vi "Get Failure Action Event.vi"(8 "error in (no error)":errorcluster, 10 "Assert VI UID":i32) -> (0 "error out":errorcluster, 3 "Failure Action Event References":T1)   [LabVIEW 2016, in "Assert API Components.lvlib" / "Log Assert Core.lvlib"]
uses:
  Log Assert Core.lvlib
  Failure Action Change Event Reference.ctl
  Failure Actions.ctl
  Assert API Components.lvlib
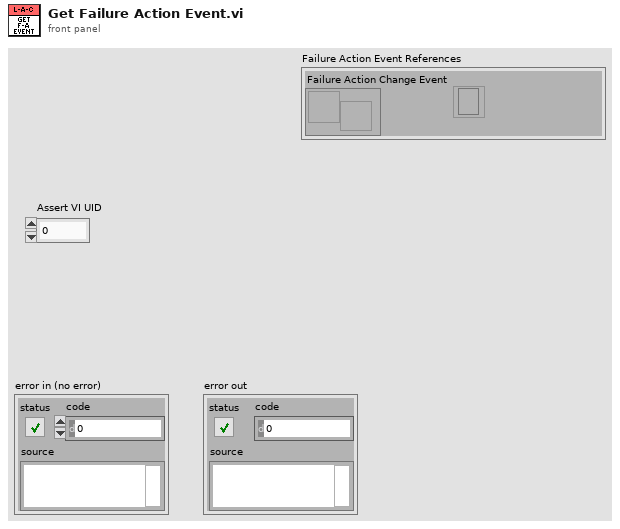
[diagram p1: front panel]
types:
  T1 = typedef "Assert API Components.lvlib/Log Assert Core.lvlib/Failure Action Change Event Reference.ctl" = cluster{"Failure Action Change Event":refnum<user-event>, "Event Registration Refnum":refnum<event-registration>}
  T2 = typedef "Assert API Components.lvlib/Failure Actions.ctl" = enum16{"None", "Log To File", "Pause Execution", "Abort Execution"}
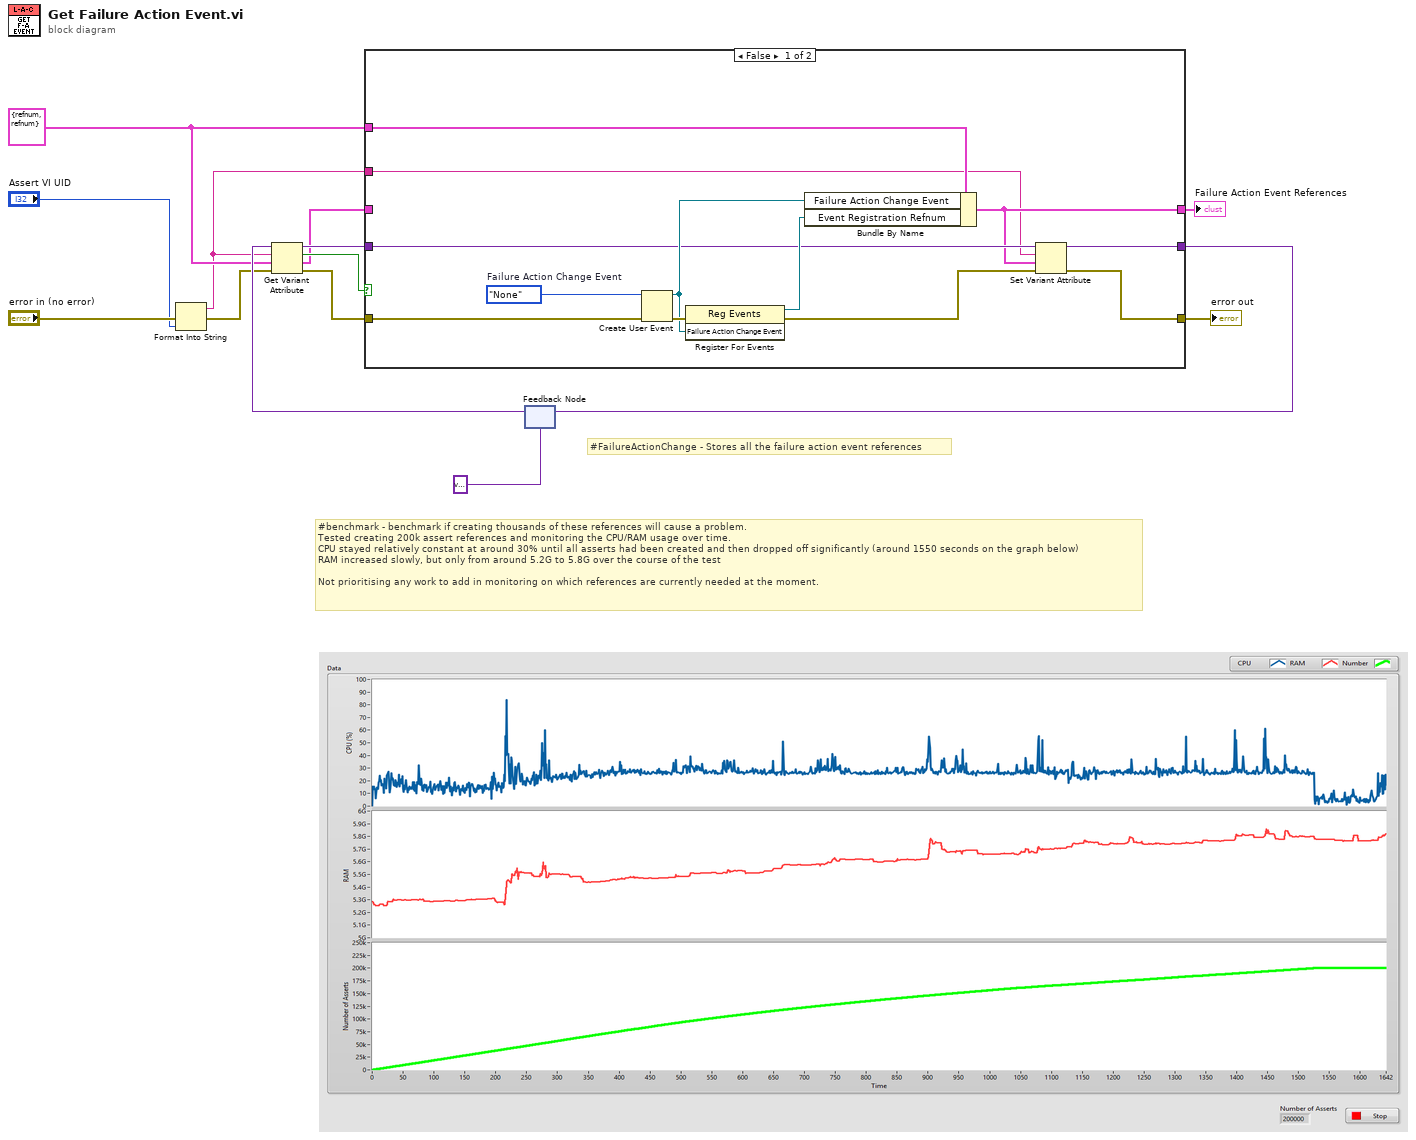
[diagram p0: block diagram]
diagram:
  w5 = T1 {"Failure Action Change Event"=refnum, "Event Registration Refnum"=refnum} ("Cluster")
  # "#benchmark - benchmark if creating thousands of these references will cause a problem. \nTested creating 200k assert references and monitoring the CPU/RAM usage over time.\nCPU stayed relatively constant at around 30% until all asserts had been created and then dropped off significantly (around 1550 seconds on the graph below)\nRAM increased slowly, but only from around 5.2G to 5.8G over the course of the test\n\nNot prioritising any work to add in monitoring on which references are currently needed at the moment."
  # "#FailureActionChange - Stores all the failure action event references"
  n1 = Format Into String(error in="error in (no error)", "Assert VI UID") -> (resulting string=w2:string, error out=w7:errorcluster)  [unwired: 2 in]
  n2 = feedback #1(variant) -> (w11:variant)
  n3 = Get Variant Attribute(Variant=w11, name=w2, default value (empty Variant)=w5, error in=w7) -> (duplicate Variant=w10:variant, found=w4:bool, value=w3:T1, error out=w8:errorcluster)
  n4 = case shown="False" w4 {
    tunnel: [w19 w29] -> w14
    tunnel: w8 -> [w25 w29]
    tunnel: w10 -> [w18 w28]
    tunnel: [w16 w27] -> w1
    tunnel: [w17 w28] -> w13
    tunnel: w5 -> [w20 _]
    tunnel: w3 -> [_ w27]
    tunnel: w2 -> [w15 _]
    frame False {
      w24 = Failure_Actions."None"  # Failure Action Change Event
      n5 = Create User Event(user event datatype=w24, error in=w25) -> (user event=w22:refnum<user-event>, error out=w23:errorcluster)
      n6 = register-events(error in=w23, w22) -> (reference out=w21:refnum<event-registration>, error out=w26:errorcluster)  [unwired: 1 in]
      n7 = Bundle By Name(cluster=w20, "Failure Action Change Event"=w22, "Event Registration Refnum"=w21) -> (w16:T1)
      n8 = Set Variant Attribute(Variant=w18, name=w15, value=w16, error in=w26) -> (Variant out=w17:variant, error out=w19:errorcluster)  [unwired: 1 out]
    }
    frame True {
    }
  }
  "error out" <- w14
  "Failure Action Event References" <- w1
  n9 = feedback-in #1(w13) -> ()
